vi "read csv file.vi"(8 "error in":errorcluster, 9 "file name":string, 10 "file path":string) -> (0 "error out":errorcluster, 2 "csv array":string[][](array[string]))   [LabVIEW 2018]
uses:
  <vilib>/Utility/file.llb/Read Delimited Spreadsheet (string).vi
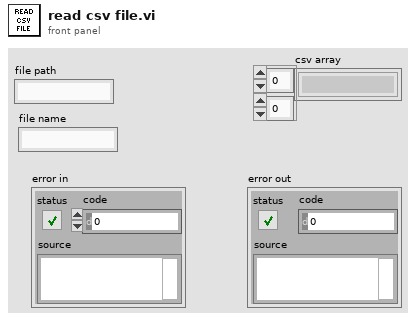
[diagram p1: front panel]
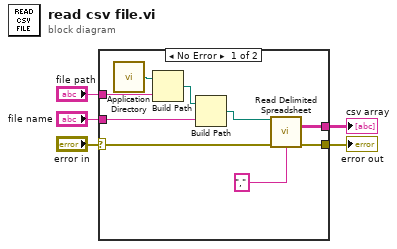
[diagram p0: block diagram]
diagram:
  n1 = case shown="No Error" "error in" {
    selector: "error in" -> [w13 w15]
    tunnel: [w12 w15] -> w3
    tunnel: [w11 _] -> w2
    tunnel: "file path" -> [w7 _]
    tunnel: "file name" -> [w6 _]
    frame No Error {
      n2 = call <vilib>:"Application Directory.vi"() -> ("Application Directory"=w10:path)
      n3 = Build Path(base path=w10, name or relative path=w7) -> (appended path=w9:path)
      n4 = Build Path(base path=w9, name or relative path=w6) -> (appended path=w8:path)
      n5 = call-poly <vilib>:"Read Delimited Spreadsheet.vi"("file path (dialog if empty)"=w8, "error in (no error)"=w13, "delimiter (\\t)"="," ("delimiter (\\t)")) -> ("all rows"=w11:string[][], "error out"=w12:errorcluster)  [unwired: 7 in, 4 out]
    }
    frame Error {
    }
  }
  "error out" <- w3
  "csv array" <- w2
